vi "Initialise.vi"(8 "error in (no error)":errorcluster, 11 "Actor in":refnum<class "Alarm Handler Actor.lvclass">) -> (0 "error out":errorcluster, 3 "Actor out":refnum<class "Alarm Handler Actor.lvclass">, 5 "Observers":cluster{"Actor":refnum<event-registration>})   [LabVIEW 2015, in "Alarm Handler Actor.lvclass"]
uses:
  Alarm Handler Actor.lvclass
  Re-use Libraries/Minimal Actor Framework/Messaging/Message/Message.lvclass
  Alarm Handler Actor.lvclass/Alarm Handler Actor.ctl
  Re-use Libraries/Utility/Utility.lvlib
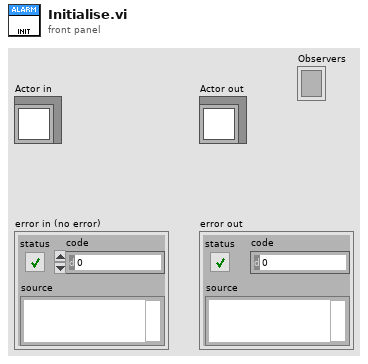
[diagram p1: front panel]
types:
  T1 = typedef "Alarm Handler Actor.lvclass/Alarm Details.ctl" = cluster{"Code":i32, "Loop":i32, "Description":string, "Severity":i32, "Clear on Ack?":bool, "Log All Events?":bool}
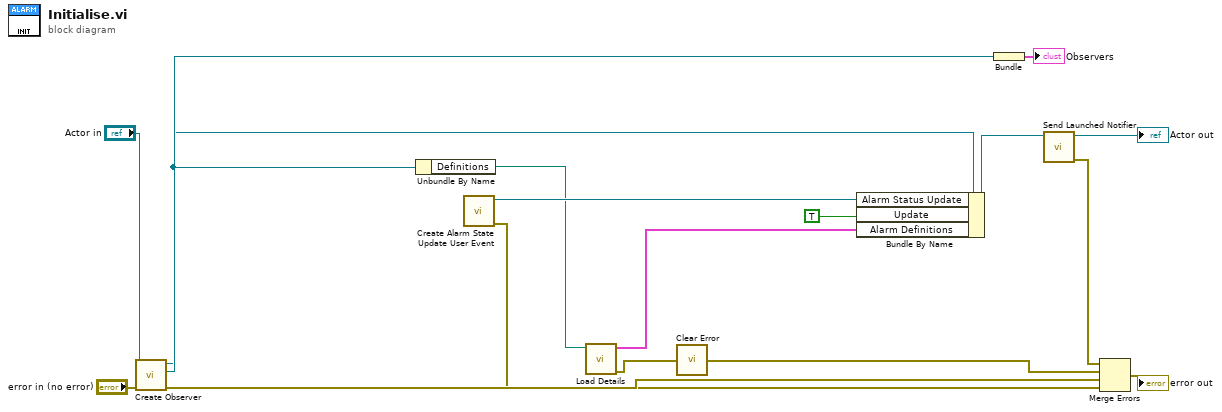
[diagram p0: block diagram]
diagram:
  n1 = call-dynamic "Create Observer.vi"("error in (no error)"="error in (no error)", "Actor in"="Actor in") -> ("error out"=w6:errorcluster, "Actor"=w9:refnum<event-registration>, "Actor out"=w8:refnum<class "Alarm Handler Actor.lvclass">)  [unwired: 7 in]
  n2 = Unbundle By Name(w8) -> ("Definitions"=w4:path)
  n3 = call "Create Alarm State Update User Event.vi"() -> ("error out"=w5:errorcluster, "Alarm State"=w11:refnum<user-event>)  [unwired: 10 in]
  n4 = call "Load Details.vi"("Alarms"=w4) -> ("error out"=w3:errorcluster, "Alarms Details"=w10:T1[])  [unwired: 9 in]
  n5 = call "Clear Error.vi"("error in (no error)"=w3) -> ("error out"=w2:errorcluster)
  n6 = Bundle By Name(cluster=w8, "Alarm Status Update"=w11, "Update"=TRUE, "Alarm Definitions"=w10) -> (w14:refnum<class "Alarm Handler Actor.lvclass">)
  n7 = Bundle("Actor"=w9) -> (→"Observers":cluster{"Actor":refnum<event-registration>})  [unwired: 1 in]
  n8 = call-dynamic "Send Launched Notifier.vi"("Actor in"=w14) -> ("error out"=w7:errorcluster, "Actor out"=→"Actor out":refnum<class "Alarm Handler Actor.lvclass">)  [unwired: 9 in]
  n9 = Merge Errors(w7, w2, w6, w5) -> (→"error out":errorcluster)
